vi "AbbyTest.vi"() -> (1 "Array":string[](array[string]), 2 "appended path":path, 3 "Refnum out":refnum<k35>)   [LabVIEW 2022 SP3]
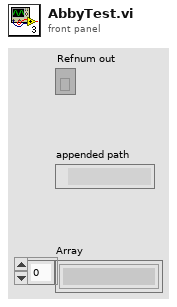
[diagram p1: front panel]
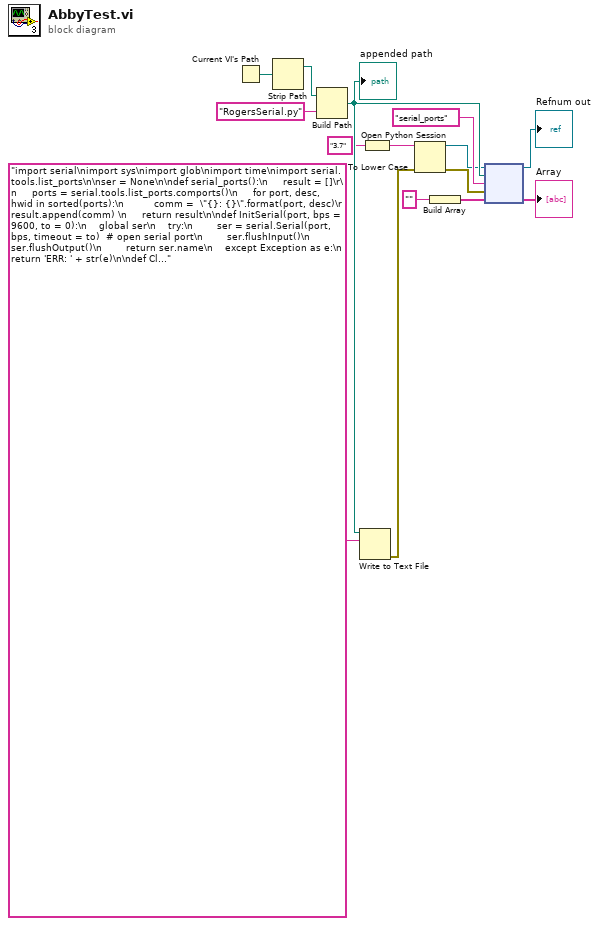
[diagram p0: block diagram]
diagram:
  n1 = Current VI's Path() -> (path=w4:path)
  n2 = Strip Path(path=w4) -> (stripped path=w3:path)  [unwired: 1 out]
  n3 = Build Path(base path=w3, name or relative path="RogersSerial.py") -> (appended path=w14:path)
  "appended path" <- w14
  n4 = Write to Text File(file (use dialog)=w14, text="import serial\nimport sys\nimport glob\nimport time\nimport serial.tools.list_ports\n\nser = None\n\ndef serial_ports():\n     result = []\r\n     ports = serial.tools.list_ports.comports()\n     for port, desc, hwid in sorted(ports):\n          comm =  \"{}: {}\".format(port, desc)\r          result.append(comm) \n     return result\n\ndef InitSerial(port, bps = 9600, to = 0):\n    global ser\n    try:\n        ser = serial.Serial(port, bps, timeout = to)  # open serial port\n        ser.flushInput()\n        ser.flushOutput()\n        return ser.name\n    except Exception as e:\n        return 'ERR: ' + str(e)\n\ndef CloseSerial():\n    return('done')\n    try:\n        ser.flush()\n        ser.close()\n        return 'done'\n    except Exception as e:\n        return 'ERR: ' + str(e)    \n\ndef WriteSerial(string):\n    try:\n        reply = ser.write(string.encode())\n        return str(reply)\n    except Exception as e:\n        return 'ERR: ' + str(e)    \n\ndef WriteBytes(data,replyLength):\n    try:\n        buffer=ser.read(ser.in_waiting)\n        reply = ser.write(bytes(data))\n        if (replyLength < 0): return []\n        return list(ser.read(replyLength))    # write bytes and get reply\n    except Exception as e:\n        return 'ERR: ' + str(e)    \n\ndef ReadSerial():\n    try:\n        reply = ''\n        if ser.in_waiting:\n            reply = ser.readline().decode()\n        return reply\n    except Exception as e:\n        return 'ERR: ' +  str(e)\n\n# note if the timeout is anything but zero it is slow") -> (error out=w6:errorcluster)  [unwired: 2 in, 2 out]
  n5 = To Lower Case(string="3.7" ("Python version")) -> (all lower case string=w9:string)
  n6 = Open Python Session(python version=w9, 3:w6) -> (session out=w2:refnum<k35>, error out=w7:errorcluster)  [unwired: 1 in]
  n7 = Build Array("" ("function name")) -> (w10:string[])
  n8 = node(w2, w14, "serial_ports" ("function name"), w7, w10) -> (→"Refnum out":refnum<k35>, →"Array":string[])  [unwired: 3 out]
